vi "SetNext.vi"(8 "error in (no error)":errorcluster, 10 "Next":refnum<class "HandlerCore.lvclass">, 11 "ErrorHandler(Handler) in":refnum<class "ErrorHandler(Handler).lvclass">) -> (0 "error out":errorcluster, 3 "ErrorHandler(Handler) out":refnum<class "ErrorHandler(Handler).lvclass">)   [LabVIEW 2014, in "Chain Of Responsibility Pattern.lvlib" / "ErrorHandler(Handler).lvclass"]
uses:
  ErrorHandler(Handler).lvclass
  HandlerCore_class/HandlerCore.lvclass
  ErrorHandler(Handler).lvclass/ErrorHandler(Handler).ctl
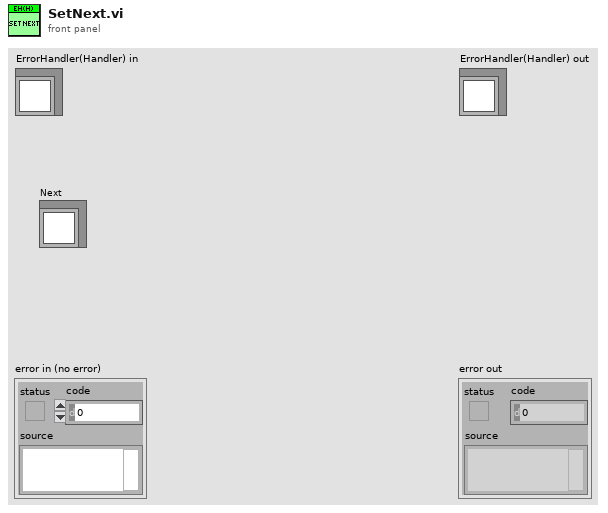
[diagram p1: front panel]
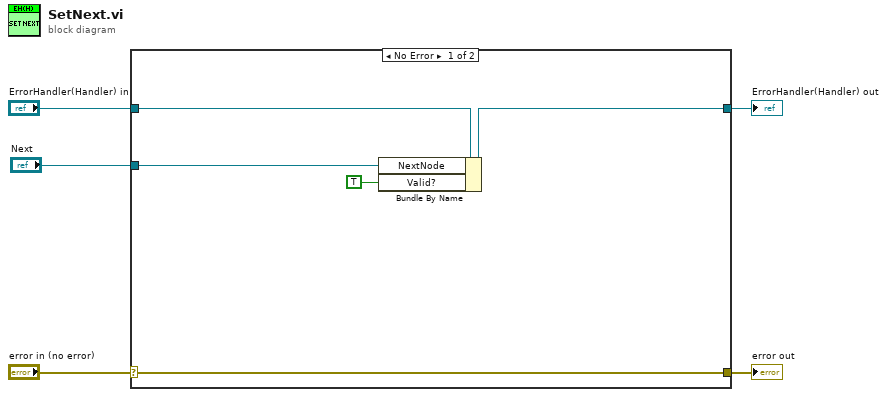
[diagram p0: block diagram]
diagram:
  n1 = case shown="No Error" "error in (no error)" {
    selector: "error in (no error)" -> [w9 w12]
    tunnel: [w9 w12] -> w4
    tunnel: [w8 w11] -> w2
    tunnel: "ErrorHandler(Handler) in" -> [w10 w11]
    tunnel: "Next" -> [w7 _]
    frame No Error {
      n2 = Bundle By Name(cluster=w10, "NextNode"=w7, "Valid?"=TRUE) -> (w8:refnum<class "ErrorHandler(Handler).lvclass">)
    }
    frame Error {
    }
  }
  "error out" <- w4
  "ErrorHandler(Handler) out" <- w2
